vi "Sine Wave.vi"(8 "error in (no error)":errorcluster, 11 "Chat Room in":refnum<class "Chat Room.lvclass">) -> (0 "error out":errorcluster, 3 "Chat Room out":refnum<class "Chat Room.lvclass">)   [LabVIEW 2018, in "Chat Room.lvlib" / "Chat Room.lvclass"]
uses:
  Chat Room.lvclass
  Chat Room.lvclass/Chat Room.ctl
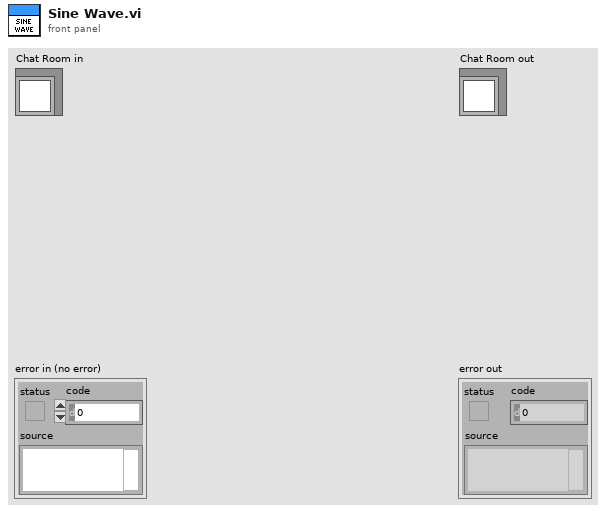
[diagram p1: front panel]
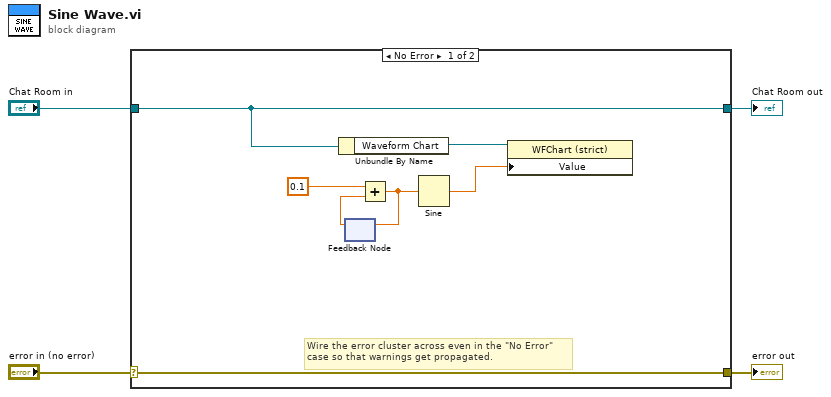
[diagram p0: block diagram]
diagram:
  n1 = case shown="No Error" "error in (no error)" {
    selector: "error in (no error)" -> [w11 w13]
    tunnel: [w11 w13] -> w3
    tunnel: [w7 w12] -> w1
    tunnel: "Chat Room in" -> [w7 w12]
    frame No Error {
      # "Wire the error cluster across even in the \"No Error\"\ncase so that warnings get propagated."
      n2 = Unbundle By Name(w7) -> ("Waveform Chart"=w6:refnum<vi>)
      n3 = feedback #1() -> (w8:dbl)  [unwired: 1 in]
      n4 = Add(x=0.1, y=w8) -> (x+y=w9:dbl)
      n5 = feedback-in #1(w9) -> ()
      n6 = Sine(x=w9) -> (sin(x)=w5:dbl)
      n7 = property class="WFChart (strict)"(reference=w6, "Value"=w5) -> ()  [unwired: 1 in, 2 out]
    }
    frame Error {
    }
  }
  "error out" <- w3
  "Chat Room out" <- w1
